vi "Read Start Order.vi"(8 "error in (no error)":errorcluster, 11 "Dependency in":refnum<class "Dependency.lvclass">) -> (0 "error out":errorcluster, 2 "Start Order":i8, 3 "Dependency out":refnum<class "Dependency.lvclass">)   [LabVIEW 2019, in "Dependency.lvclass"]
doc: "JKI State Machine Objects (SMO) 1.3.0.56\nJKI - JKI\nCopyright (c) 2017, JKI"
uses:
  Dependency.lvclass
  Dependency.lvclass/Dependency.ctl
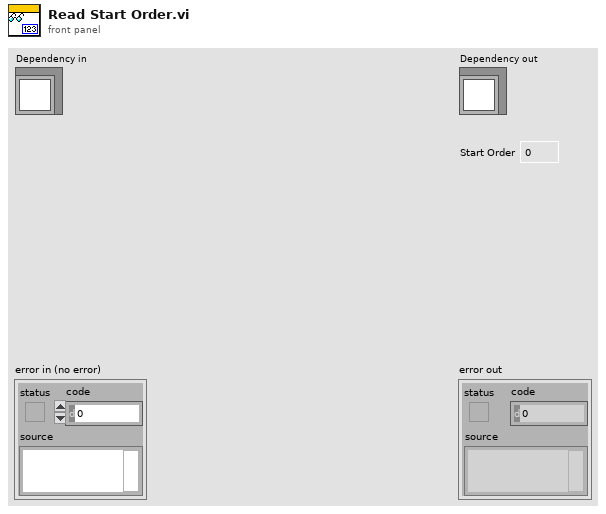
[diagram p1: front panel]
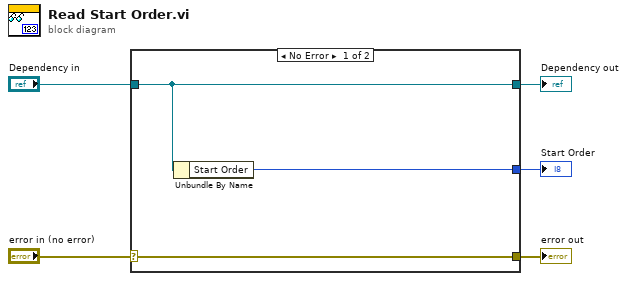
[diagram p0: block diagram]
diagram:
  n1 = case shown="No Error" "error in (no error)" {
    selector: "error in (no error)" -> [w8 w9]
    tunnel: [w8 w9] -> w4
    tunnel: [w7 w10] -> w2
    tunnel: "Dependency in" -> [w7 w10]
    tunnel: [w6 _] -> w1
    frame No Error {
      n2 = Unbundle By Name(w7) -> ("Start Order"=w6:i8)
    }
    frame Error {
    }
  }
  "error out" <- w4
  "Dependency out" <- w2
  "Start Order" <- w1
